vi "gStatus.vi"() -> ()   [LabVIEW 2024]
uses:
  Type Definitions.llb/OperationMode.ctt
  Type Definitions.llb/3 way Status.ctl
panel:
  in  "Exposure":T1=1 items=["N.A.", "OK", "Busy", "Done"]
  in  "Sleep?":bool
  in  "PDA":T1 items=["N.A.", "OK", "Busy", "Done"]
  in  "Operation Mode":T2
  in  "Exp Index":u32
  in  "Saving":T1 items=["N.A.", "OK", "Busy", "Done"]
  in  "Plotting":T1 items=["N.A.", "OK", "Busy", "Done"]
  in  "Buffer":T1 items=["N.A.", "OK", "Busy", "Done"]
  in  "CCD":T1 items=["N.A.", "OK", "Busy", "Done"]
  in  "Ev(nm)":T1 items=["N.A.", "OK", "Busy", "Done"]
  in  "T(K)":T1 items=["N.A.", "OK", "Busy", "Done"]
  in  "H(T)":T1 items=["N.A.", "OK", "Busy", "Done"]
  # "Status Global Controls"
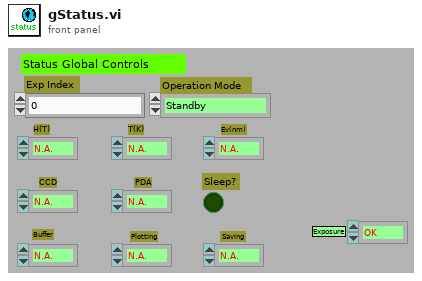
[diagram p1: front panel]
types:
  T1 = typedef "3 way Status.ctl" = u8
  T2 = typedef "OperationMode.ctt" = enum16{"Standby", "CCD Single Shot", "CCD Sequence Shots", "CCD Custom Shots", "CCD Reference Shot", "Step Scanning ", "Time Scanning", "NML Data Acquisition"}
diagram:
